vi "Scripting_RemoveSubViAndFixWires.vi"(1 "MainViPath/ViRef/BlockDiagramRef":variant, 2 "SubVIToRemove":path, 3 "SaveVIBeforeRemove(False)":bool, 5 "error in (no error)":errorcluster, 6 "AppRef":refnum<vi>) -> (19 "error out":errorcluster)   [LabVIEW 2020]
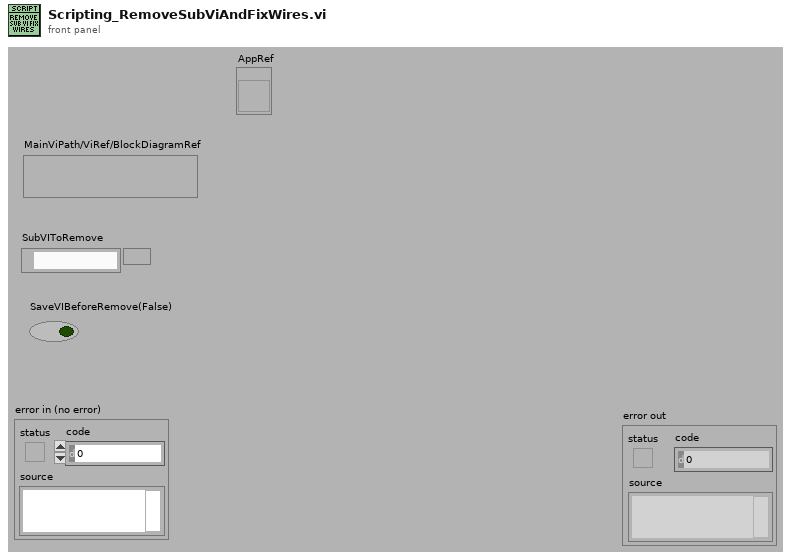
[diagram p1: front panel]
types:
  T1 = cluster{"ViRef":refnum<vi>, "BlockDiagramRef":refnum<vi>, "SubVIOwner":refnum<vi>, "SubVI":refnum<vi>}
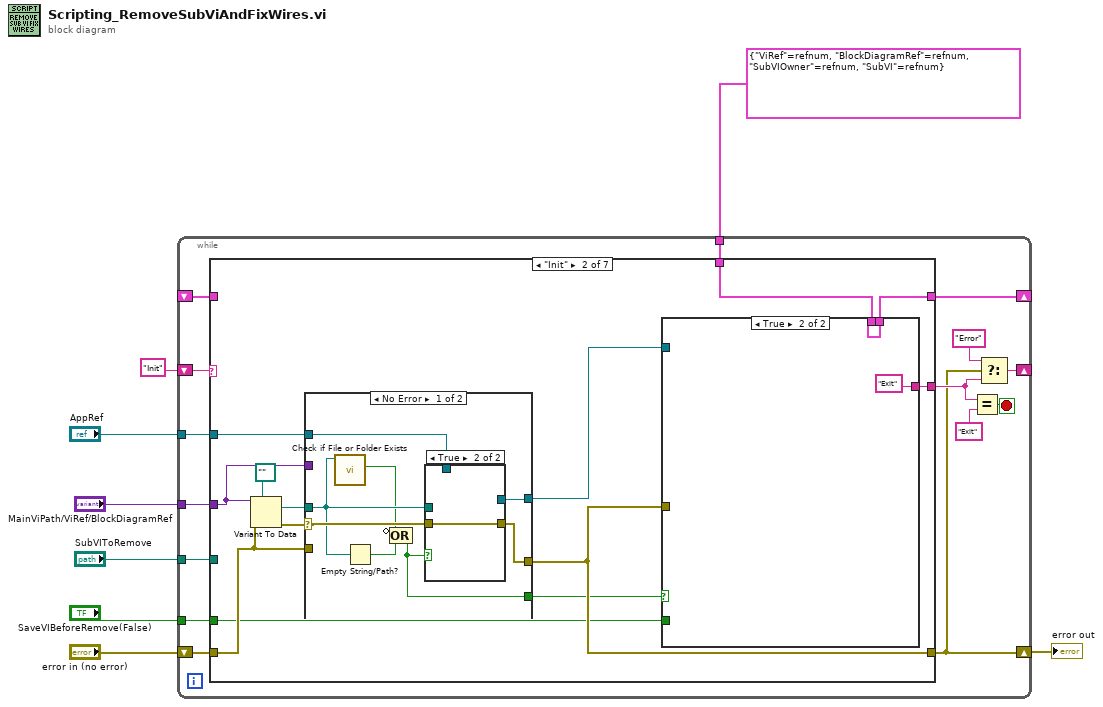
[diagram p0: block diagram]
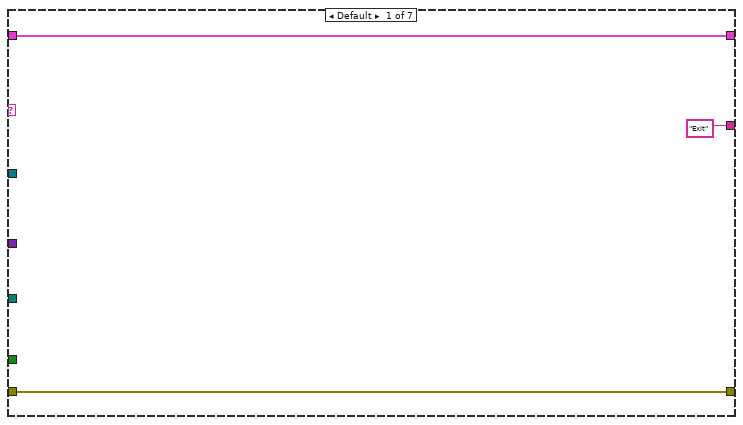
[diagram p2: hidden frame]
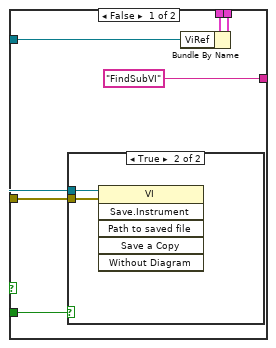
[diagram p3: hidden frame]
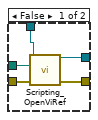
[diagram p5: hidden frame]
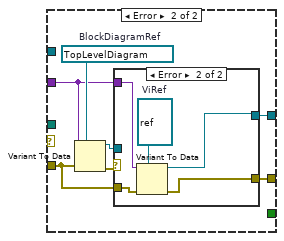
[diagram p6: hidden frame]
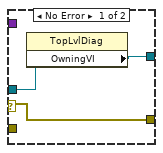
[diagram p7: hidden frame]
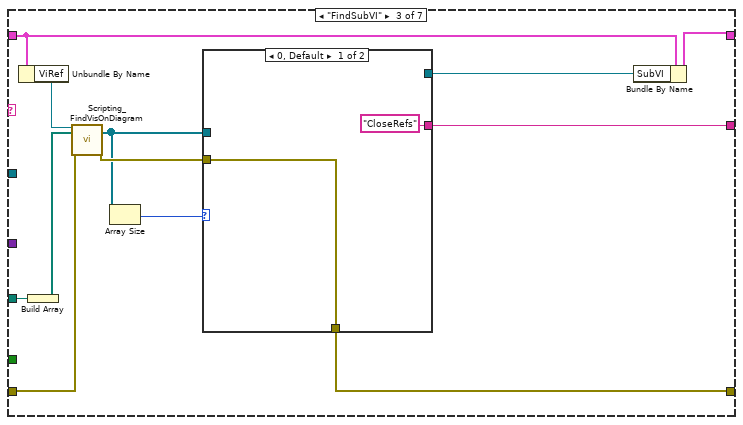
[diagram p8: hidden frame]
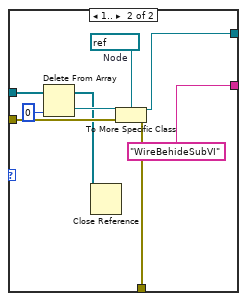
[diagram p9: hidden frame]
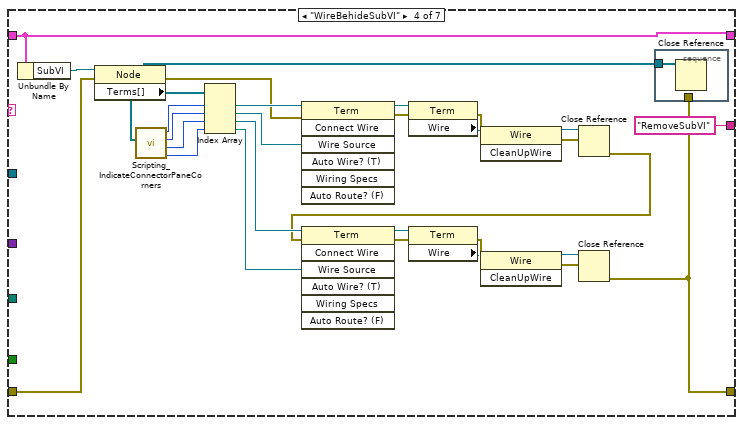
[diagram p10: hidden frame]
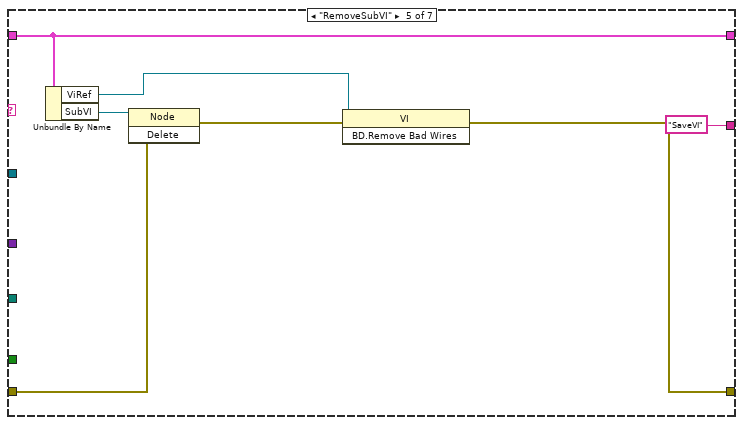
[diagram p11: hidden frame]
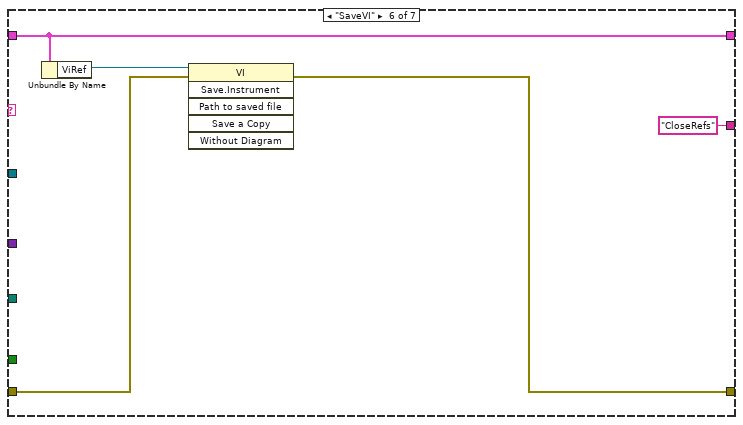
[diagram p12: hidden frame]
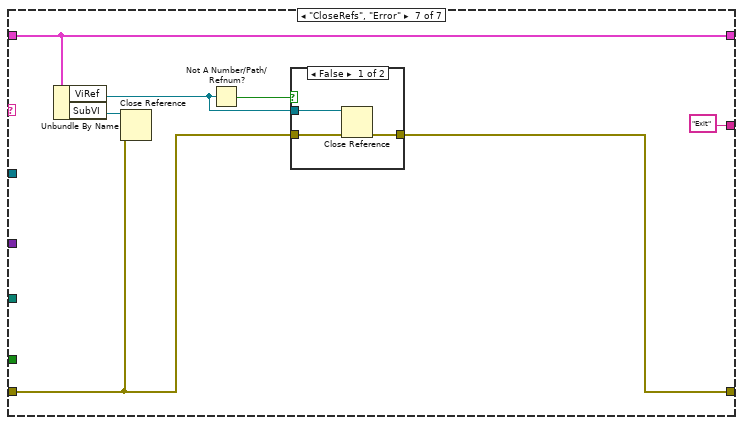
[diagram p13: hidden frame]
diagram:
  n1 = while {
    shift-right: [w16] -> w6
    shift-left: "error in (no error)" -> [w23]
    shift-right: [w21] -> _
    shift-left: "Init" -> [w22]
    shift-right: [w15] -> _
    shift-left: _ -> [w14]
    tunnel: "MainViPath/ViRef/BlockDiagramRef" -> [w13]
    tunnel: "SubVIToRemove" -> [w12]
    tunnel: T1 {"ViRef"=refnum, "BlockDiagramRef"=refnum, "SubVIOwner"=refnum, "SubVI"=refnum} -> [w11]
    tunnel: "SaveVIBeforeRemove(False)" -> [w10]
    tunnel: "AppRef" -> [w9]
    stop <- w20 stop-if-true
    n2 = case shown="\"Init\"" w22 {
      tunnel: w23 -> [w26 w34 w87 w122 w136 w141 w143]
      tunnel: [w26 w30 w83 w102 w132 w140 w145] -> w16
      tunnel: ["Exit" w39 w79 "RemoveSubVI" "SaveVI" "CloseRefs" "Exit"] -> w17
      tunnel: [w24 w35 w85 w128 w134 w139 w148] -> w15
      tunnel: w14 -> [w24 _ w86 w128 w134 w139 w148]
      tunnel: w13 -> [_ w32 _ _ _ _ _]
      tunnel: w12 -> [_ _ w90 _ _ _ _]
      tunnel: w11 -> [_ w33 _ _ _ _ _]
      tunnel: w10 -> [_ w29 _ _ _ _ _]
      tunnel: w9 -> [_ w28 _ _ _ _ _]
      frame Default {
      }
      frame "Init" {
        n3 = Variant To Data(error in=w34, type=path "", Variant=w32) -> (data=w36:path, error out=w37:errorcluster)
        n4 = case shown="No Error" w37 {
          selector: w37 -> [w57 _]
          tunnel: w34 -> [_ w67]
          tunnel: w36 -> [w53 _]
          tunnel: [w55 w64] -> w31
          tunnel: [w56 w66] -> w30
          tunnel: w32 -> [_ w65]
          tunnel: w28 -> [w54 _]
          tunnel: [w50 _] -> w27
          frame No Error {
            n5 = call <vilib>:"Check if File or Folder Exists.vi"("path"=w53) -> ("file or folder exists?"=w52:bool)  [unwired: 8 in, 2 out]
            n6 = Empty String/Path?(string/path=w53) -> (empty?=w51:bool)
            n7 = Compound Arithmetic op=OR(invert w52, w51) -> (w50:bool)
            n8 = case shown="True" w50 {
              tunnel: w57 -> [w62 w63]
              tunnel: [w61 w63] -> w56
              tunnel: [w60 _] -> w55
              tunnel: w54 -> [w59 _]
              tunnel: w53 -> [w58 _]
              frame False {
                n9 = call "Scripting_OpenViRef.vi"("error in"=w62, "ViPath/ViName/Viref"=w58, "AppRef"=w59) -> ("error out"=w61:errorcluster, "vi reference"=w60:refnum<vi>)  [unwired: 6 in, 1 out]
              }
              frame True {
              }
            }
          }
          frame Error {
            w70 = refnum<vi> refnum  # BlockDiagramRef
            n10 = Variant To Data(error in=w67, type=w70, Variant=w65) -> (data=w68:refnum<vi>, error out=w69:errorcluster)
            n11 = case shown="Error" w69 {
              selector: w69 -> [w73 _]
              tunnel: w68 -> [w72 _]
              tunnel: w67 -> [_ w78]
              tunnel: [w73 w74] -> w66
              tunnel: w65 -> [_ w76]
              tunnel: [w71 w75] -> w64
              frame No Error {
                n12 = property class="TopLvlDiag"(reference=w72) -> ("OwningVI"=w71:refnum<vi>)  [unwired: 1 in, 2 out]
              }
              frame Error {
                w77 = refnum<vi> refnum  # ViRef
                n13 = Variant To Data(error in=w78, type=w77, Variant=w76) -> (data=w75:refnum<vi>, error out=w74:errorcluster)
              }
            }
          }
        }
        n14 = case shown="True" w27 {
          tunnel: ["FindSubVI" "Exit"] -> w39
          tunnel: [w44 w49] -> w35
          tunnel: w33 -> [w43 w49]
          tunnel: w31 -> [w42 _]
          tunnel: w30 -> [w41 _]
          tunnel: w29 -> [w40 _]
          frame False {
            n15 = case shown="True" w40 {
              tunnel: w42 -> [_ w47]
              tunnel: w41 -> [_ w46]
              frame False {
              }
              frame True {
                n16 = invoke class="VI" method="Save.Instrument"(reference=w47, error in=w46) -> ()  [unwired: 4 in, 6 out]
              }
            }
            n17 = Bundle By Name(cluster=w43, "ViRef"=w42) -> (w44:T1)
          }
          frame True {
          }
        }
      }
      frame "FindSubVI" {
        n18 = Unbundle By Name(w86) -> ("ViRef"=w88:refnum<vi>)
        n19 = Build Array(w90) -> (w89:path[])
        n20 = call "Scripting_FindVisOnDiagram.vi"("ViRef"=w88, "VIsToSerachFor/ViName"=w89, "error in (no error)"=w87) -> ("VisFound"=w81:refnum<vi>[], "error out"=w82:errorcluster)  [unwired: 15 in]
        n21 = Array Size(array=w81) -> (size(s)=w80:i32)
        n22 = case shown="0, Default" w80 {
          tunnel: [_ w100] -> w84
          tunnel: [w91 w99] -> w83
          tunnel: w82 -> [w91 w98]
          tunnel: w81 -> [_ w96]
          tunnel: ["CloseRefs" "WireBehideSubVI"] -> w79
          frame 0, Default {
          }
          frame 1.. {
            w101 = refnum<vi> refnum  # Node
            n23 = Delete From Array(array=w96, index=0) -> (deleted portion=w95:refnum<vi>, array with subset deleted=w93:refnum<vi>[])  [unwired: 1 in]
            n24 = Close Reference(reference=w93) -> ()  [unwired: 1 in, 1 out]
            n25 = To More Specific Class(target class=w101, reference=w95, error in=w98) -> (specific class reference=w100:refnum<vi>, error out=w99:errorcluster)
          }
        }
        n26 = Bundle By Name(cluster=w86, "SubVI"=w84) -> (w85:T1)
      }
      frame "WireBehideSubVI" {
        n27 = Unbundle By Name(w128) -> ("SubVI"=w121:refnum<vi>)
        n28 = property class="Node"(reference=w121, error in=w122) -> (error out=w123:errorcluster, "Terms[]"=w120:refnum<vi>[])  [unwired: 1 out]
        n29 = call "Scripting_IndicateConnectorPaneCorners.vi"("Terminals[]"=w120) -> ("RightLower"=w116:i32, "LeftLower"=w117:i32, "RightTop"=w118:i32, "LeftTop"=w119:i32)  [unwired: 7 in]
        n30 = Index Array(array=w120, index #1=w119, index #2=w118, index #3=w117, index #4=w116) -> (element #1=w127:refnum<vi>, element #2=w126:refnum<vi>, element #3=w125:refnum<vi>, element #4=w124:refnum<vi>)
        n31 = invoke class="Term" method="Connect Wire"(reference=w127, error in=w123, "Wire Source"=w126) -> (reference out=w115:refnum<vi>, error out=w114:errorcluster)  [unwired: 4 in, 5 out]
        n32 = property class="Term"(reference=w115, error in=w114) -> (error out=w110:errorcluster, "Wire"=w113:refnum<vi>)  [unwired: 1 out]
        n33 = invoke class="Wire" method="CleanUpWire"(reference=w113, error in=w110) -> (reference out=w112:refnum<vi>, error out=w111:errorcluster)  [unwired: 1 in, 1 out]
        n34 = Close Reference(reference=w112, error in (no error)=w111) -> (error out=w109:errorcluster)
        n35 = invoke class="Term" method="Connect Wire"(reference=w125, error in=w109, "Wire Source"=w124) -> (reference out=w104:refnum<vi>, error out=w103:errorcluster)  [unwired: 4 in, 5 out]
        n36 = property class="Term"(reference=w104, error in=w103) -> (error out=w108:errorcluster, "Wire"=w105:refnum<vi>)  [unwired: 1 out]
        n37 = invoke class="Wire" method="CleanUpWire"(reference=w105, error in=w108) -> (reference out=w106:refnum<vi>, error out=w107:errorcluster)  [unwired: 1 in, 1 out]
        n38 = Close Reference(reference=w106, error in (no error)=w107) -> (error out=w102:errorcluster)
        n39 = stacked-sequence {
          tunnel: w120 -> [w130]
          tunnel: w102 -> [_]
          frame #0 {
            n40 = Close Reference(reference=w130) -> ()  [unwired: 1 in, 1 out]
          }
        }
      }
      frame "RemoveSubVI" {
        n41 = Unbundle By Name(w134) -> ("ViRef"=w133:refnum<vi>, "SubVI"=w137:refnum<vi>)
        n42 = invoke class="Node" method="Delete"(reference=w137, error in=w136) -> (error out=w131:errorcluster)  [unwired: 1 in, 2 out]
        n43 = invoke class="VI" method="BD.Remove Bad Wires"(reference=w133, error in=w131) -> (error out=w132:errorcluster)  [unwired: 1 in, 2 out]
      }
      frame "SaveVI" {
        n44 = Unbundle By Name(w139) -> ("ViRef"=w142:refnum<vi>)
        n45 = invoke class="VI" method="Save.Instrument"(reference=w142, error in=w141) -> (error out=w140:errorcluster)  [unwired: 4 in, 5 out]
      }
      frame "CloseRefs", "Error" {
        n46 = Unbundle By Name(w148) -> ("ViRef"=w146:refnum<vi>, "SubVI"=w144:refnum<vi>)
        n47 = Close Reference(reference=w144, error in (no error)=w143) -> ()  [unwired: 1 out]
        n48 = Not A Number/Path/Refnum?(number/path/refnum=w146) -> (NaN/Path/Refnum?=w147:bool)
        n49 = case shown="False" w147 {
          tunnel: w143 -> [w152 w153]
          tunnel: w146 -> [w151 _]
          tunnel: [w150 w153] -> w145
          frame False {
            n50 = Close Reference(reference=w151, error in (no error)=w152) -> (error out=w150:errorcluster)
          }
          frame True {
          }
        }
      }
    }
    n51 = Equal?(x=w17, y="Exit") -> (x = y?=w20:bool)
    n52 = Select(t="Error", s=w16, f=w17) -> (s? t:f=w21:string)
  }
  "error out" <- w6
